vi "Manager.vi"() -> ()   [LabVIEW 2021, in "CIFPluginManager.lvclass"]
uses:
  CIFPluginManager.lvclass
  CIFPluginManager.lvclass/CIFPluginManager.ctl
  <vilib>/CIF Foundation/CIF Core/CIFUtilities/CIFLogs/CIFLogs.lvlib
panel:
  in  "stop":bool
  # "This is displayed for debugging.  In final release this will not be displayed."
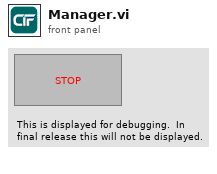
[diagram p1: front panel]
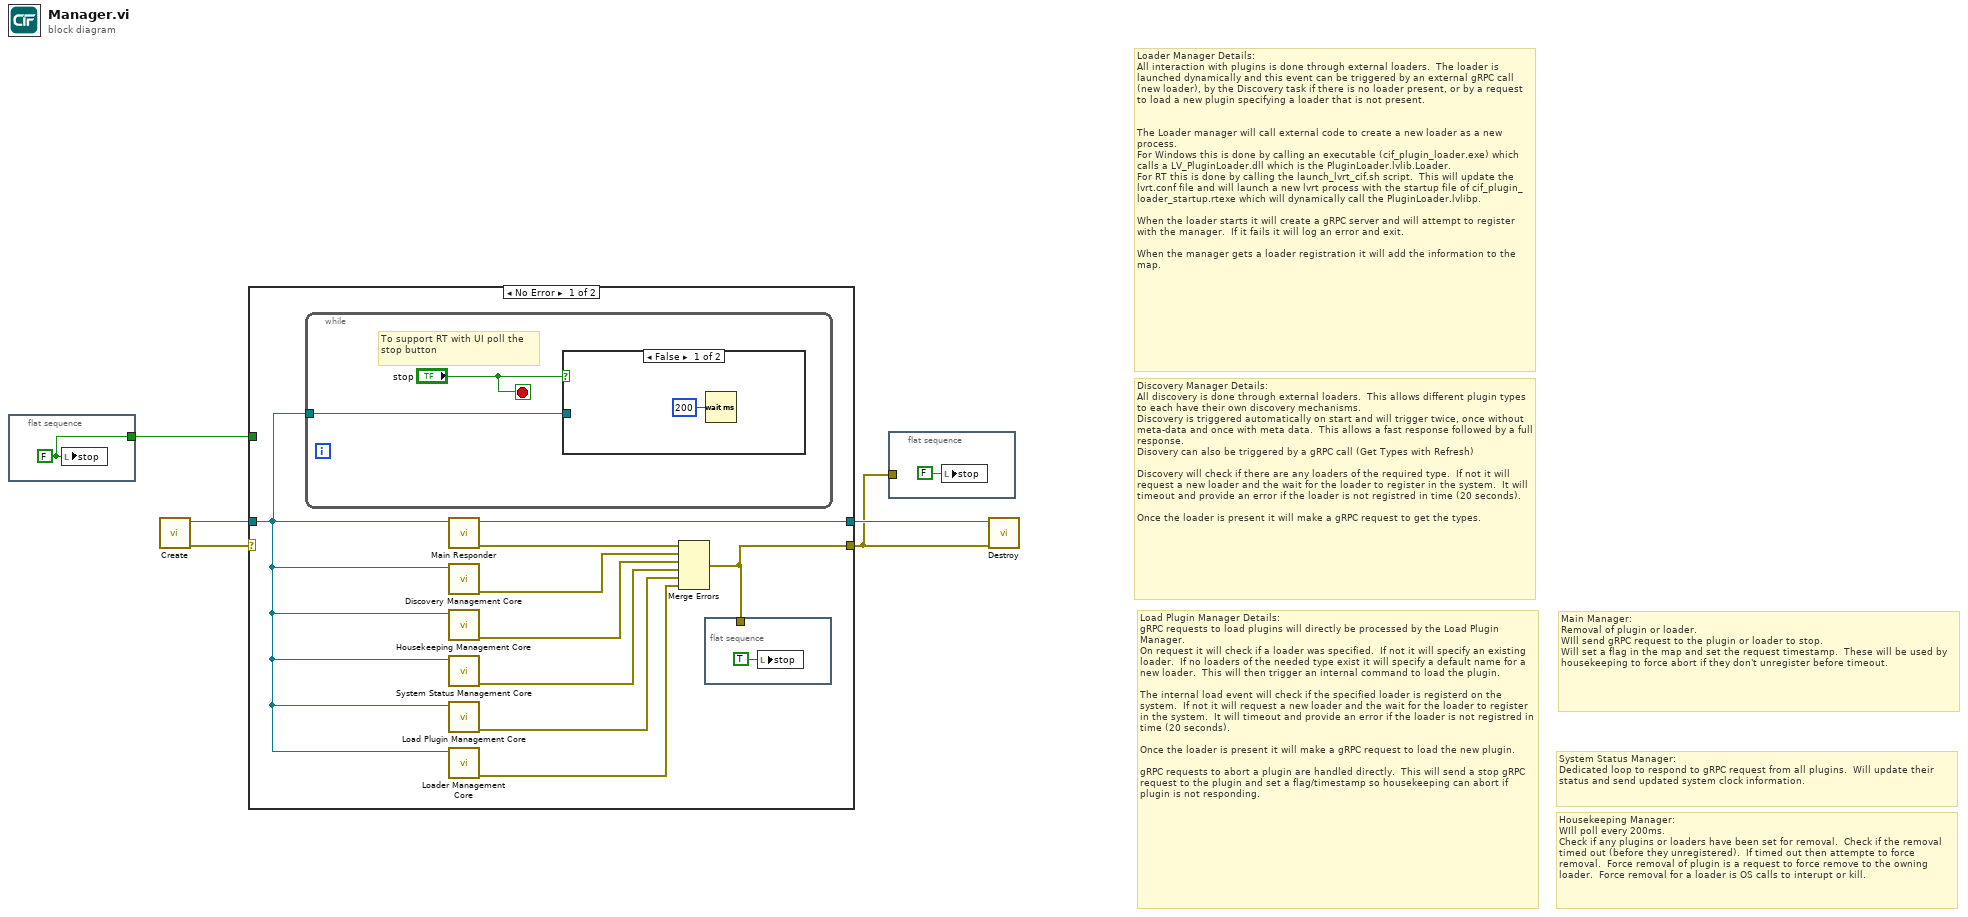
[diagram p0: block diagram]
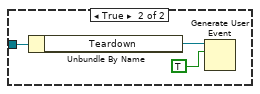
[diagram p2: hidden frame]
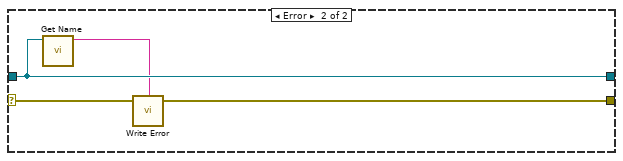
[diagram p3: hidden frame]
diagram:
  # "Main Manager:\nRemoval of plugin or loader.\nWIll send gRPC request to the plugin or loader to stop.\nWill set a flag in the map and set the request timestamp.  These will be used by housekeeping to force abort if they don't unregister before timeout."
  # "System Status Manager:\nDedicated loop to respond to gRPC request from all plugins.  Will update their status and send updated system clock information."
  # "Housekeeping Manager:\nWIll poll every 200ms.\nCheck if any plugins or loaders have been set for removal.  Check if the removal timed out (before they unregistered).  If timed out then attempte to force removal.  Force removal of plugin is a request to force remove to the owning loader.  Force removal for a loader is OS calls to interupt or kill."
  # "Load Plugin Manager Details:\ngRPC requests to load plugins will directly be processed by the Load Plugin Manager.\nOn request it will check if a loader was specified.  If not it will specify an existing loader.  If no loaders of the needed type exist it will specify a default name for a new loader.  This will then trigger an internal command to load the plugin.\n\nThe internal load event will check if the specified loader is registerd on the system.  If not it will request a new loader and the wait for the loader to register in the system.  It will timeout and provide an error if the loader is not registred in time (20 seconds).\n\nOnce the loader is present it will make a gRPC request to load the new plugin.\n\ngRPC requests to abort a plugin are handled directly.  This will send a stop gRPC request to the plugin and set a flag/timestamp so housekeeping can abort if plugin is not responding."
  # "Discovery Manager Details:\nAll discovery is done through external loaders.  This allows different plugin types to each have their own discovery mechanisms.\nDiscovery is triggered automatically on start and will trigger twice, once without meta-data and once with meta data.  This allows a fast response followed by a full response.\nDisovery can also be triggered by a gRPC call (Get Types with Refresh)\n\nDiscovery will check if there are any loaders of the required type.  If not it will request a new loader and the wait for the loader to register in the system.  It will timeout and provide an error if the loader is not registred in time (20 seconds).\n\nOnce the loader is present it will make a gRPC request to get the types."
  # "Loader Manager Details:\nAll interaction with plugins is done through external loaders.  The loader is launched dynamically and this event can be triggered by an external gRPC call (new loader), by the Discovery task if there is no loader present, or by a request to load a new plugin specifying a loader that is not present.\n\n\nThe Loader manager will call external code to create a new loader as a new process.  \nFor Windows this is done by calling an executable (cif_plugin_loader.exe) which calls a LV_PluginLoader.dll which is the PluginLoader.lvlib.Loader.   \nFor RT this is done by calling the launch_lvrt_cif.sh script.  This will update the lvrt.conf file and will launch a new lvrt process with the startup file of cif_plugin_loader_startup.rtexe which will dynamically call the PluginLoader.lvlibp.\n\nWhen the loader starts it will create a gRPC server and will attempt to register with the manager.  If it fails it will log an error and exit.\n\nWhen the manager gets a loader registration it will add the information to the map."
  n1 = flat-sequence {
    tunnel: [w6] -> w2
    frame #0 {
      w6 = FALSE ("stop")
      n2 = local write "stop"(w6) -> ()
    }
  }
  n3 = call "Create.vi"() -> ("error out"=w4:errorcluster, "Plugin Manager out"=w5:refnum<class "CIFPluginManager.lvclass">)  [unwired: 10 in]
  n4 = case shown="No Error" w4 {
    selector: w4 -> [_ w26]
    tunnel: w5 -> [w8 w24]
    tunnel: [w15 w24] -> w3
    tunnel: [w9 w25] -> w1
    tunnel: w2 -> [_ _]
    frame No Error {
      n5 = while {
        tunnel: w8 -> [w18]
        stop <- "stop" stop-if-true
        # "To support RT with UI poll the stop button"
        n6 = case shown="False" "stop" {
          tunnel: w18 -> [_ w20]
          frame False {
            n7 = Wait (ms)(milliseconds to wait=u32 200) -> ()  [unwired: 1 out]
          }
          frame True {
            n8 = Unbundle By Name(w20) -> ("Teardown"=w21:refnum<user-event>)
            n9 = Generate User Event(user event=w21, event data cluster=TRUE ("event data")) -> ()  [unwired: 2 in, 2 out]
          }
        }
      }
      n10 = call "Main Responder.vi"("CIFPluginManager in"=w8) -> ("error out"=w14:errorcluster, "Plugin Manager out"=w15:refnum<class "CIFPluginManager.lvclass">)  [unwired: 9 in]
      n11 = call "Discovery Management Core.vi"("CIFPluginManager in"=w8) -> ("error out"=w13:errorcluster)  [unwired: 10 in]
      n12 = call "Housekeeping Management Core.vi"("CIFPluginManager in"=w8) -> ("error out"=w12:errorcluster)  [unwired: 10 in]
      n13 = call "System Status Management Core.vi"("CIFPluginManager in"=w8) -> ("error out"=w10:errorcluster)  [unwired: 10 in]
      n14 = call "Load Plugin Management Core.vi"("CIFPluginManager in"=w8) -> ("error out"=w11:errorcluster)  [unwired: 10 in]
      n15 = call "Loader Management Core.vi"("CIFPluginManager in"=w8) -> ("error out"=w7:errorcluster)  [unwired: 10 in]
      n16 = Merge Errors(w14, w13, w12, w10, w11, w7) -> (w9:errorcluster)
      n17 = flat-sequence {
        tunnel: w9 -> [_]
        frame #0 {
          n18 = local write "stop"(TRUE ("stop")) -> ()
        }
      }
    }
    frame Error {
      n19 = call "Get Name.vi"("CIFPluginManager in"=w24) -> ("Name"=w23:string)  [unwired: 10 in]
      n20 = call <vilib>:"Write Error.vi"("error in (no error)"=w26, "Plugin Name"=w23) -> ("cleared error"=w25:errorcluster)  [unwired: 2 in]
    }
  }
  n21 = flat-sequence {
    tunnel: w1 -> [_]
    frame #0 {
      n22 = local write "stop"(FALSE ("stop")) -> ()
    }
  }
  n23 = call "Destroy.vi"("error in (no error)"=w1, "Plugin Manager in"=w3) -> ()  [unwired: 9 in, 1 out]
